vi "Find Nearest Prime Number.vi"(10 "start number":u32) -> (2 "prime number":u32)   [LabVIEW 2021]
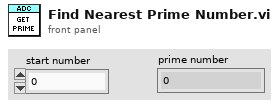
[diagram p1: front panel]
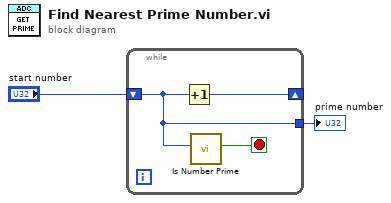
[diagram p0: block diagram]
diagram:
  n1 = while {
    shift-right: [w5] -> _
    shift-left: "start number" -> [w3]
    tunnel: [w3] -> w1
    stop <- w4 stop-if-true
    n2 = Increment(x=w3) -> (x+1=w5:u32)
    n3 = call "Is Number Prime.vi"("number"=w3) -> ("is prime"=w4:bool)  [unwired: 10 in]
  }
  "prime number" <- w1
